vi "Branch Follower.vi"() -> ()   [LabVIEW 2013]
panel:
  out "In Range?":bool
  in  "Enable Output":bool
  out "Loop Counter":i32
  in  "Stop Button":bool
  in  "Update Rate (ms)":u32=100
  in  "Axis Intercept":dbl=23659.0 format="%.4g"
  in  "Slope":dbl=0.0017 format="%.4e"
  out "Output Position":i32
  out "Output Position (dbl)":dbl
  out "Input Wavelength":dbl format="%.4g"
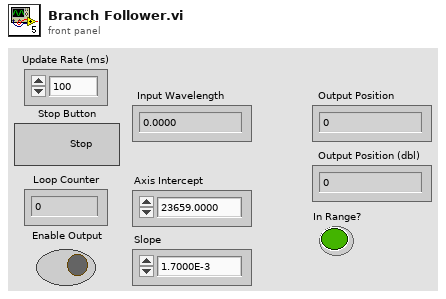
[diagram p1: front panel]
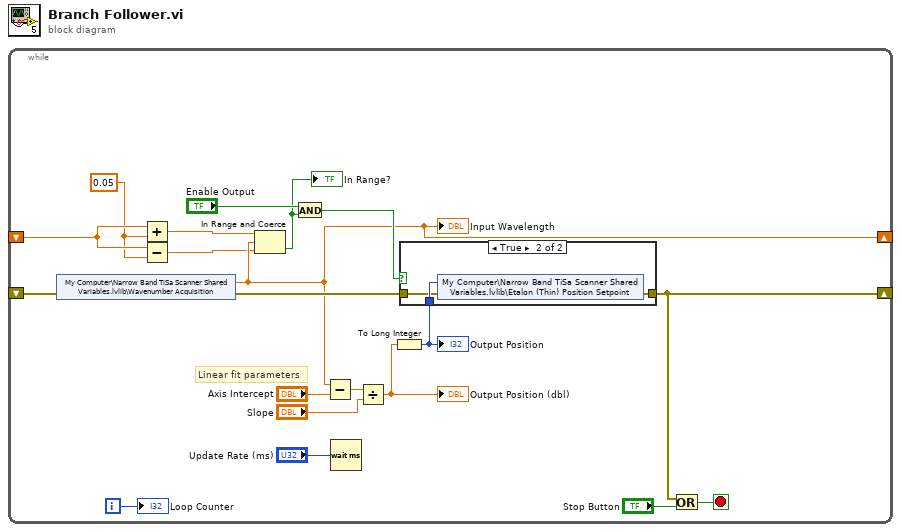
[diagram p0: block diagram]
diagram:
  n1 = while {
    shift-right: [w11] -> _
    shift-left: _ -> [w12]
    shift-right: [w5] -> _
    shift-left: _ -> [w4]
    i -> [w15]
    stop <- w9 stop-if-true
    w3 = 0.05
    # "Linear fit parameters"
    n2 = shared-variable "My Computer\\Narrow Band TiSa Scanner Shared Variables.lvlib\\Wavenumber Acquisition"(error in=w12) -> (w5:dbl, error out=w13:errorcluster)
    "Input Wavelength" <- w5
    n3 = Add(x=w4, y=w3) -> (x+y=w2:dbl)
    n4 = Subtract(x=w4, y=w3) -> (x-y=w1:dbl)
    n5 = In Range and Coerce(upper limit=w2, x=w5, lower limit=w1) -> (In Range?=w7:bool)  [unwired: 1 out]
    "In Range?" <- w7
    n6 = And(x="Enable Output", y=w7) -> (x .and. y?=w6:bool)
    n7 = Subtract(x=w5, y="Axis Intercept") -> (x-y=w18:dbl)
    n8 = Wait (ms)(milliseconds to wait="Update Rate (ms)") -> ()  [unwired: 1 out]
    n9 = Divide(x=w18, y="Slope") -> (x/y=w17:dbl)
    "Output Position (dbl)" <- w17
    n10 = To Long Integer(number=w17) -> (32bit integer=w14:i32)
    "Output Position" <- w14
    n11 = case shown="True" w6 {
      tunnel: w14 -> [_ w24]
      tunnel: w13 -> [w21 w23]
      tunnel: [w21 w22] -> w11
      frame False {
      }
      frame True {
        n12 = shared-variable "My Computer\\Narrow Band TiSa Scanner Shared Variables.lvlib\\Etalon (Thin) Position Setpoint"(w24, error in=w23) -> (error out=w22:errorcluster)
      }
    }
    n13 = Or(x=w11, y="Stop Button") -> (x .or. y?=w9:bool)
    "Loop Counter" <- w15
  }
